vi "Call_Block_plug_ins.vi"(0 "Per Block Plug Ins":string[](array[string])) -> ()   [LabVIEW 2017]
uses:
  Globals/Dynamic_call_global.ph.vi
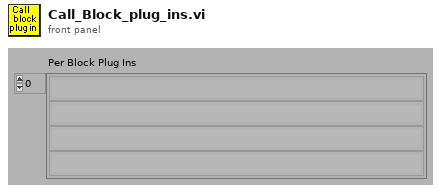
[diagram p1: front panel]
types:
  T1 = enum32{"Invalid", "Standard", "Closed", "Hidden", "Minimized", "Maximized"}
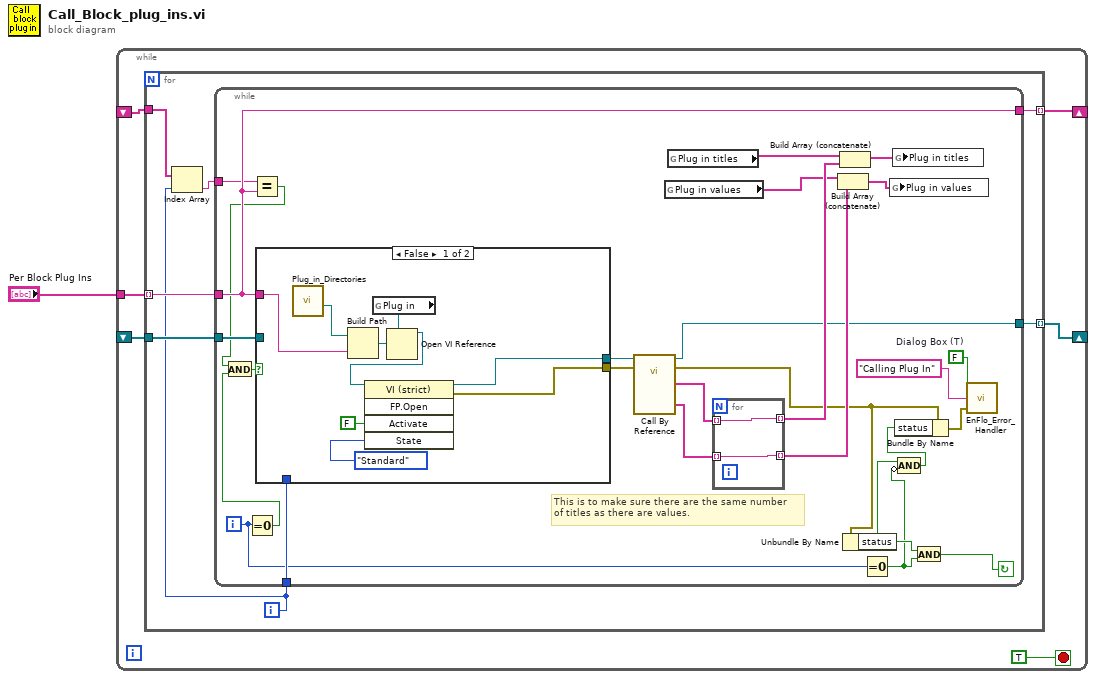
[diagram p0: block diagram]
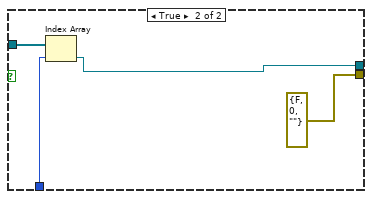
[diagram p2: hidden frame]
diagram:
  n1 = while {
    tunnel: "Per Block Plug Ins" -> [w7]
    shift-right: [w6] -> _
    shift-left: _ -> [w5]
    shift-right: [w3] -> _
    shift-left: _ -> [w2]
    stop <- TRUE stop-if-true
    n2 = for {
      tunnel: w7 -> [w14] mode=indexing
      tunnel: [w13] -> w6 mode=indexing
      tunnel: w5 -> [w12]
      tunnel: [w11] -> w3 mode=indexing
      tunnel: w2 -> [w9]
      i -> [w10]
      n3 = Index Array(array=w9, index=w10) -> (element=w8:string)
      n4 = while {
        tunnel: w14 -> [w23]
        tunnel: [w35] -> w13
        tunnel: w10 -> [w34]
        tunnel: w12 -> [w33]
        tunnel: [w23] -> w11
        tunnel: w8 -> [w22]
        i -> [w24]
        stop <- w30 continue-if-true
        w32 = FALSE  # Dialog Box (T)
        # "This is to make sure there are the same number\nof titles as there are values."
        n5 = Equal To 0?(x=w24) -> (x = 0?=w20:bool)
        n6 = Equal?(x=w22, y=w23) -> (x = y?=w19:bool)
        n7 = And(x=w19, y=w20) -> (x .and. y?=w21:bool)
        n8 = case shown="False" w21 {
          tunnel: [w42 errorcluster {"status"=FALSE, "code"=0, "source"=""} ("error out")] -> w37
          tunnel: [w43 w52] -> w36
          tunnel: w23 -> [w47 _]
          tunnel: w34 -> [_ w54]
          tunnel: w33 -> [_ w53]
          frame False {
            n9 = call "Plug_in_Directories.vi"() -> ("Per Block"=w50:path)  [unwired: 2 in, 4 out]
            n10 = Build Path(base path=w50, name or relative path=w47) -> (appended path=w48:path)
            n11 = global read "Dynamic_call_global.ph.vi" "Plug in"() -> (w49:refnum<vi>)
            n12 = Open VI Reference(type specifier VI Refnum (for type only)=w49, vi path=w48) -> (vi reference=w46:refnum<vi>)  [unwired: 2 in, 3 out]
            n13 = invoke class="VI (strict)" method="FP.Open"(reference=w46, "Activate"=FALSE ("Activate?"), "State"=T1."Standard") -> (reference out=w43:refnum<vi>, error out=w42:errorcluster)  [unwired: 2 in, 3 out]
          }
          frame True {
            n14 = Index Array(array=w53, index=w54) -> (element=w52:refnum<vi>)
          }
        }
        n15 = call-by-ref "?"(reference=w36, error in=w37) -> (reference out=w35:refnum<vi>, error out=w29:errorcluster, "Plug in titles"=w40:string[], "Plug in values"=w38:string[])  [unwired: 6 in]
        n16 = global read "Dynamic_call_global.ph.vi" "Plug in values"() -> (w18:string[])
        n17 = global read "Dynamic_call_global.ph.vi" "Plug in titles"() -> (w17:string[])
        n18 = for {
          tunnel: [w56] -> w41 mode=indexing
          tunnel: w40 -> [w56] mode=indexing
          tunnel: [w55] -> w39 mode=indexing
          tunnel: w38 -> [w55] mode=indexing
        }
        n19 = Build Array (concatenate)(w18, w39) -> (w16:string[])
        n20 = Build Array (concatenate)(w17, w41) -> (w15:string[])
        n21 = Unbundle By Name(w29) -> ("status"=w27:bool)
        n22 = Equal To 0?(x=w24) -> (x = 0?=w26:bool)
        n23 = global write "Dynamic_call_global.ph.vi" "Plug in values"(w16) -> ()
        n24 = global write "Dynamic_call_global.ph.vi" "Plug in titles"(w15) -> ()
        n25 = Compound Arithmetic op=AND(w27, invert w26) -> (w25:bool)
        n26 = Bundle By Name(cluster=w29, "status"=w25) -> (w28:errorcluster)
        n27 = And(x=w27, y=w26) -> (x .and. y?=w30:bool)
        n28 = call "EnFlo_Error_Handler.vi"("error in (no error)"=w28, "Error Type"="Calling Plug In", "Dialog Box (T)"=w32) -> ()  [unwired: 3 out]
      }
    }
  }
